vi "ReadCurrAD.vi"(6 "time out":u32, 10 "类型":u32(ring)=4 items=["PCI5121"=1, "PCI9810"=2, "USBCAN1"=3, "USBCAN2"=4, "PCI9820"=5, "CAN232"=6, "PCI5110"=7, "CANLite(mini)"=8, "ISA9620"=9, "ISA5420"=10, "PC104CAN"=11, "CANET"=17, "DNP9810"=13, "USBCAN-E-U"=20, "USBCAN-2E-U"=21], 12 "设备索引":u32(ring) items=["0", "1", "2", "3", "4", "5", "6", "7", "8", "9", "10", "11", "12", "13", "14", "15", ""], 16 "CAN路数":u32(ring) items=["0", "1"]) -> (20 "set ok?":bool, 23 "AD":u16)   [LabVIEW 2013]
uses:
  AutoBurn/Settings/ControlCAN.dll
panel:
  out "VCI_CAN_OBJ_T":T1 {"ID" format="%x"}
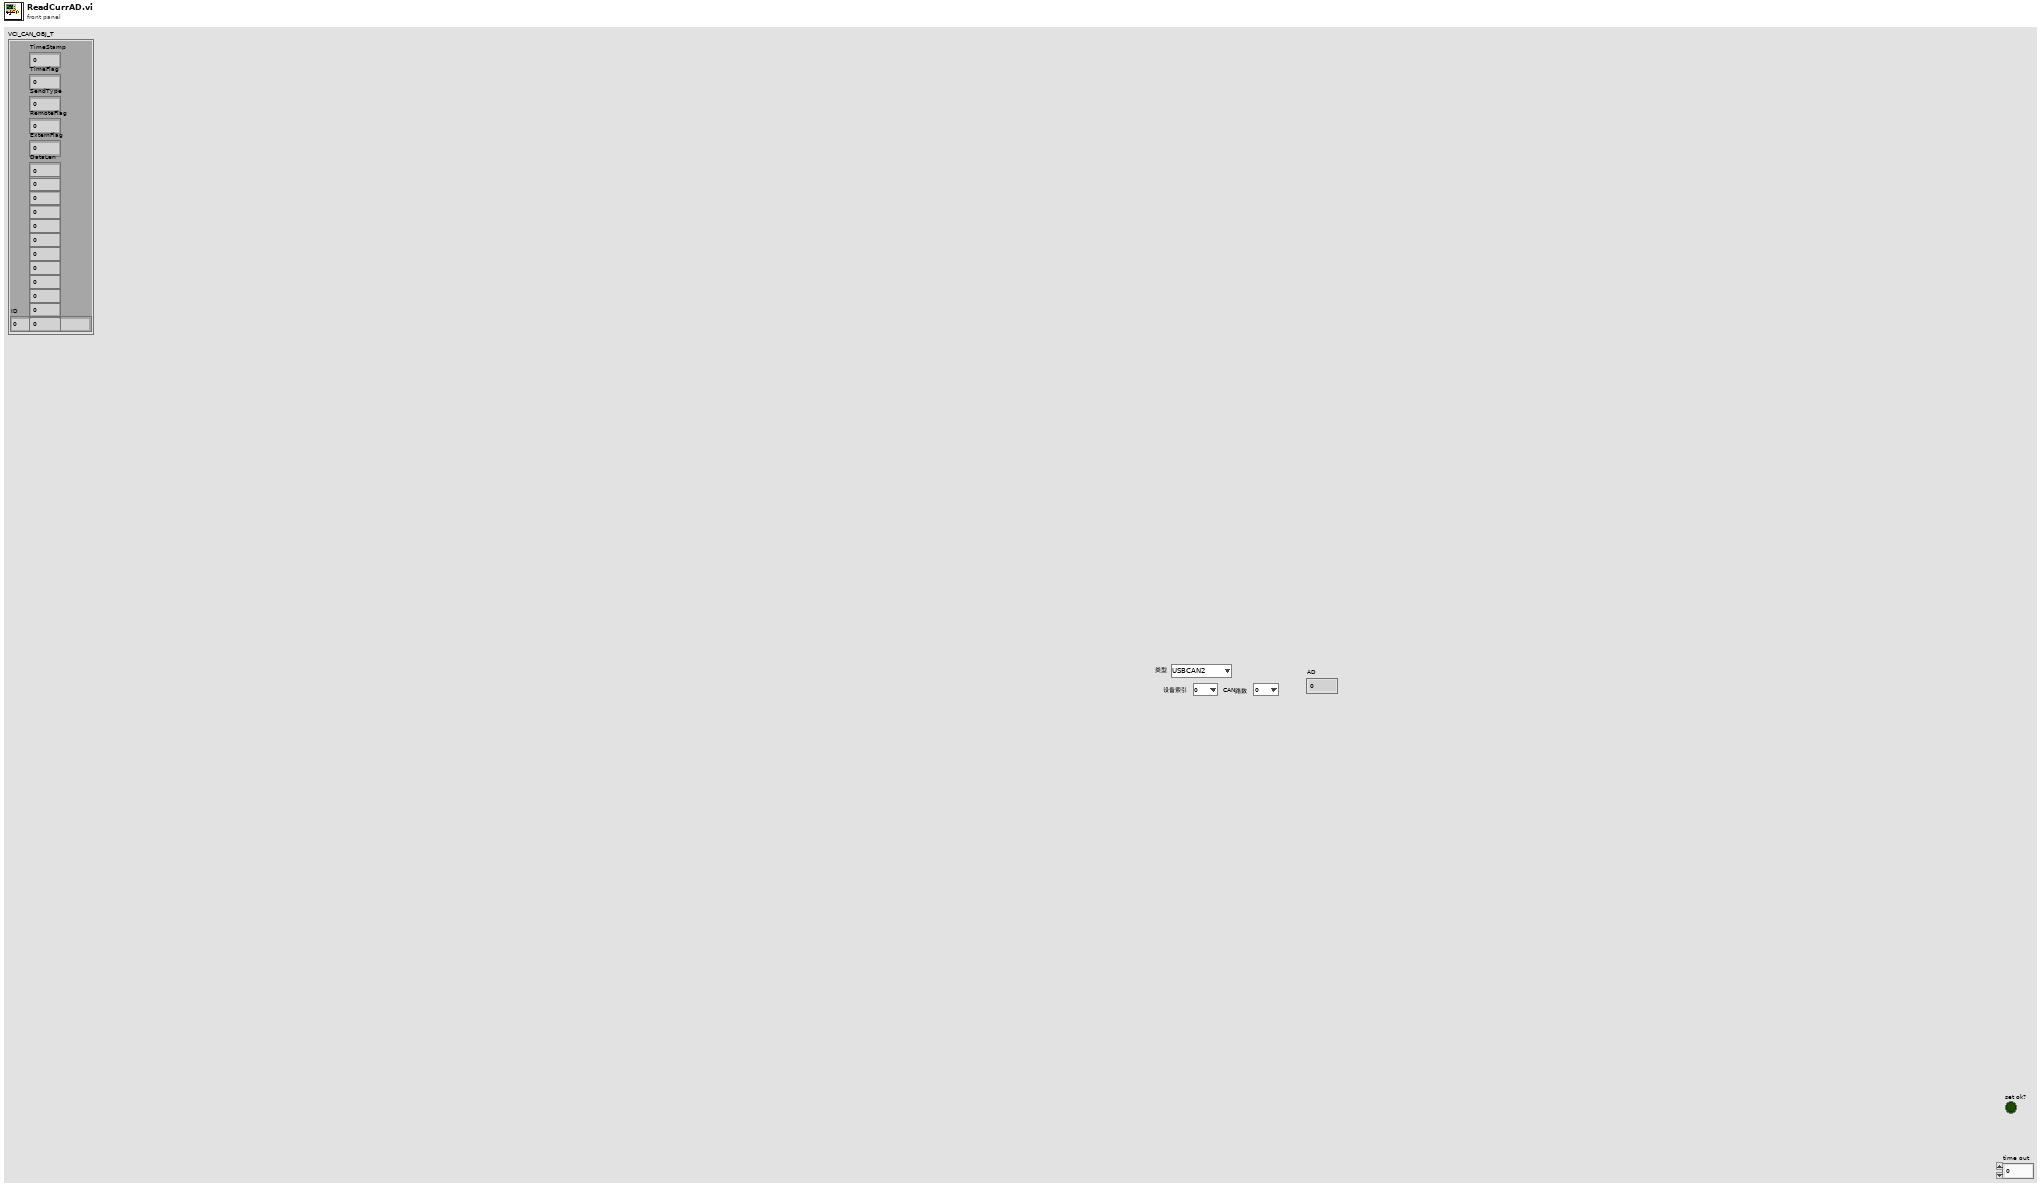
[diagram p1: front panel]
types:
  T1 = cluster{"ID":u32, "TimeStamp":u32, "TimeFlag":u8, "SendType":u8, "RemoteFlag":u8, "ExternFlag":u8, "DataLen":u8, u8, u8, u8, u8, u8, u8, u8, u8, u8, u8, u8}
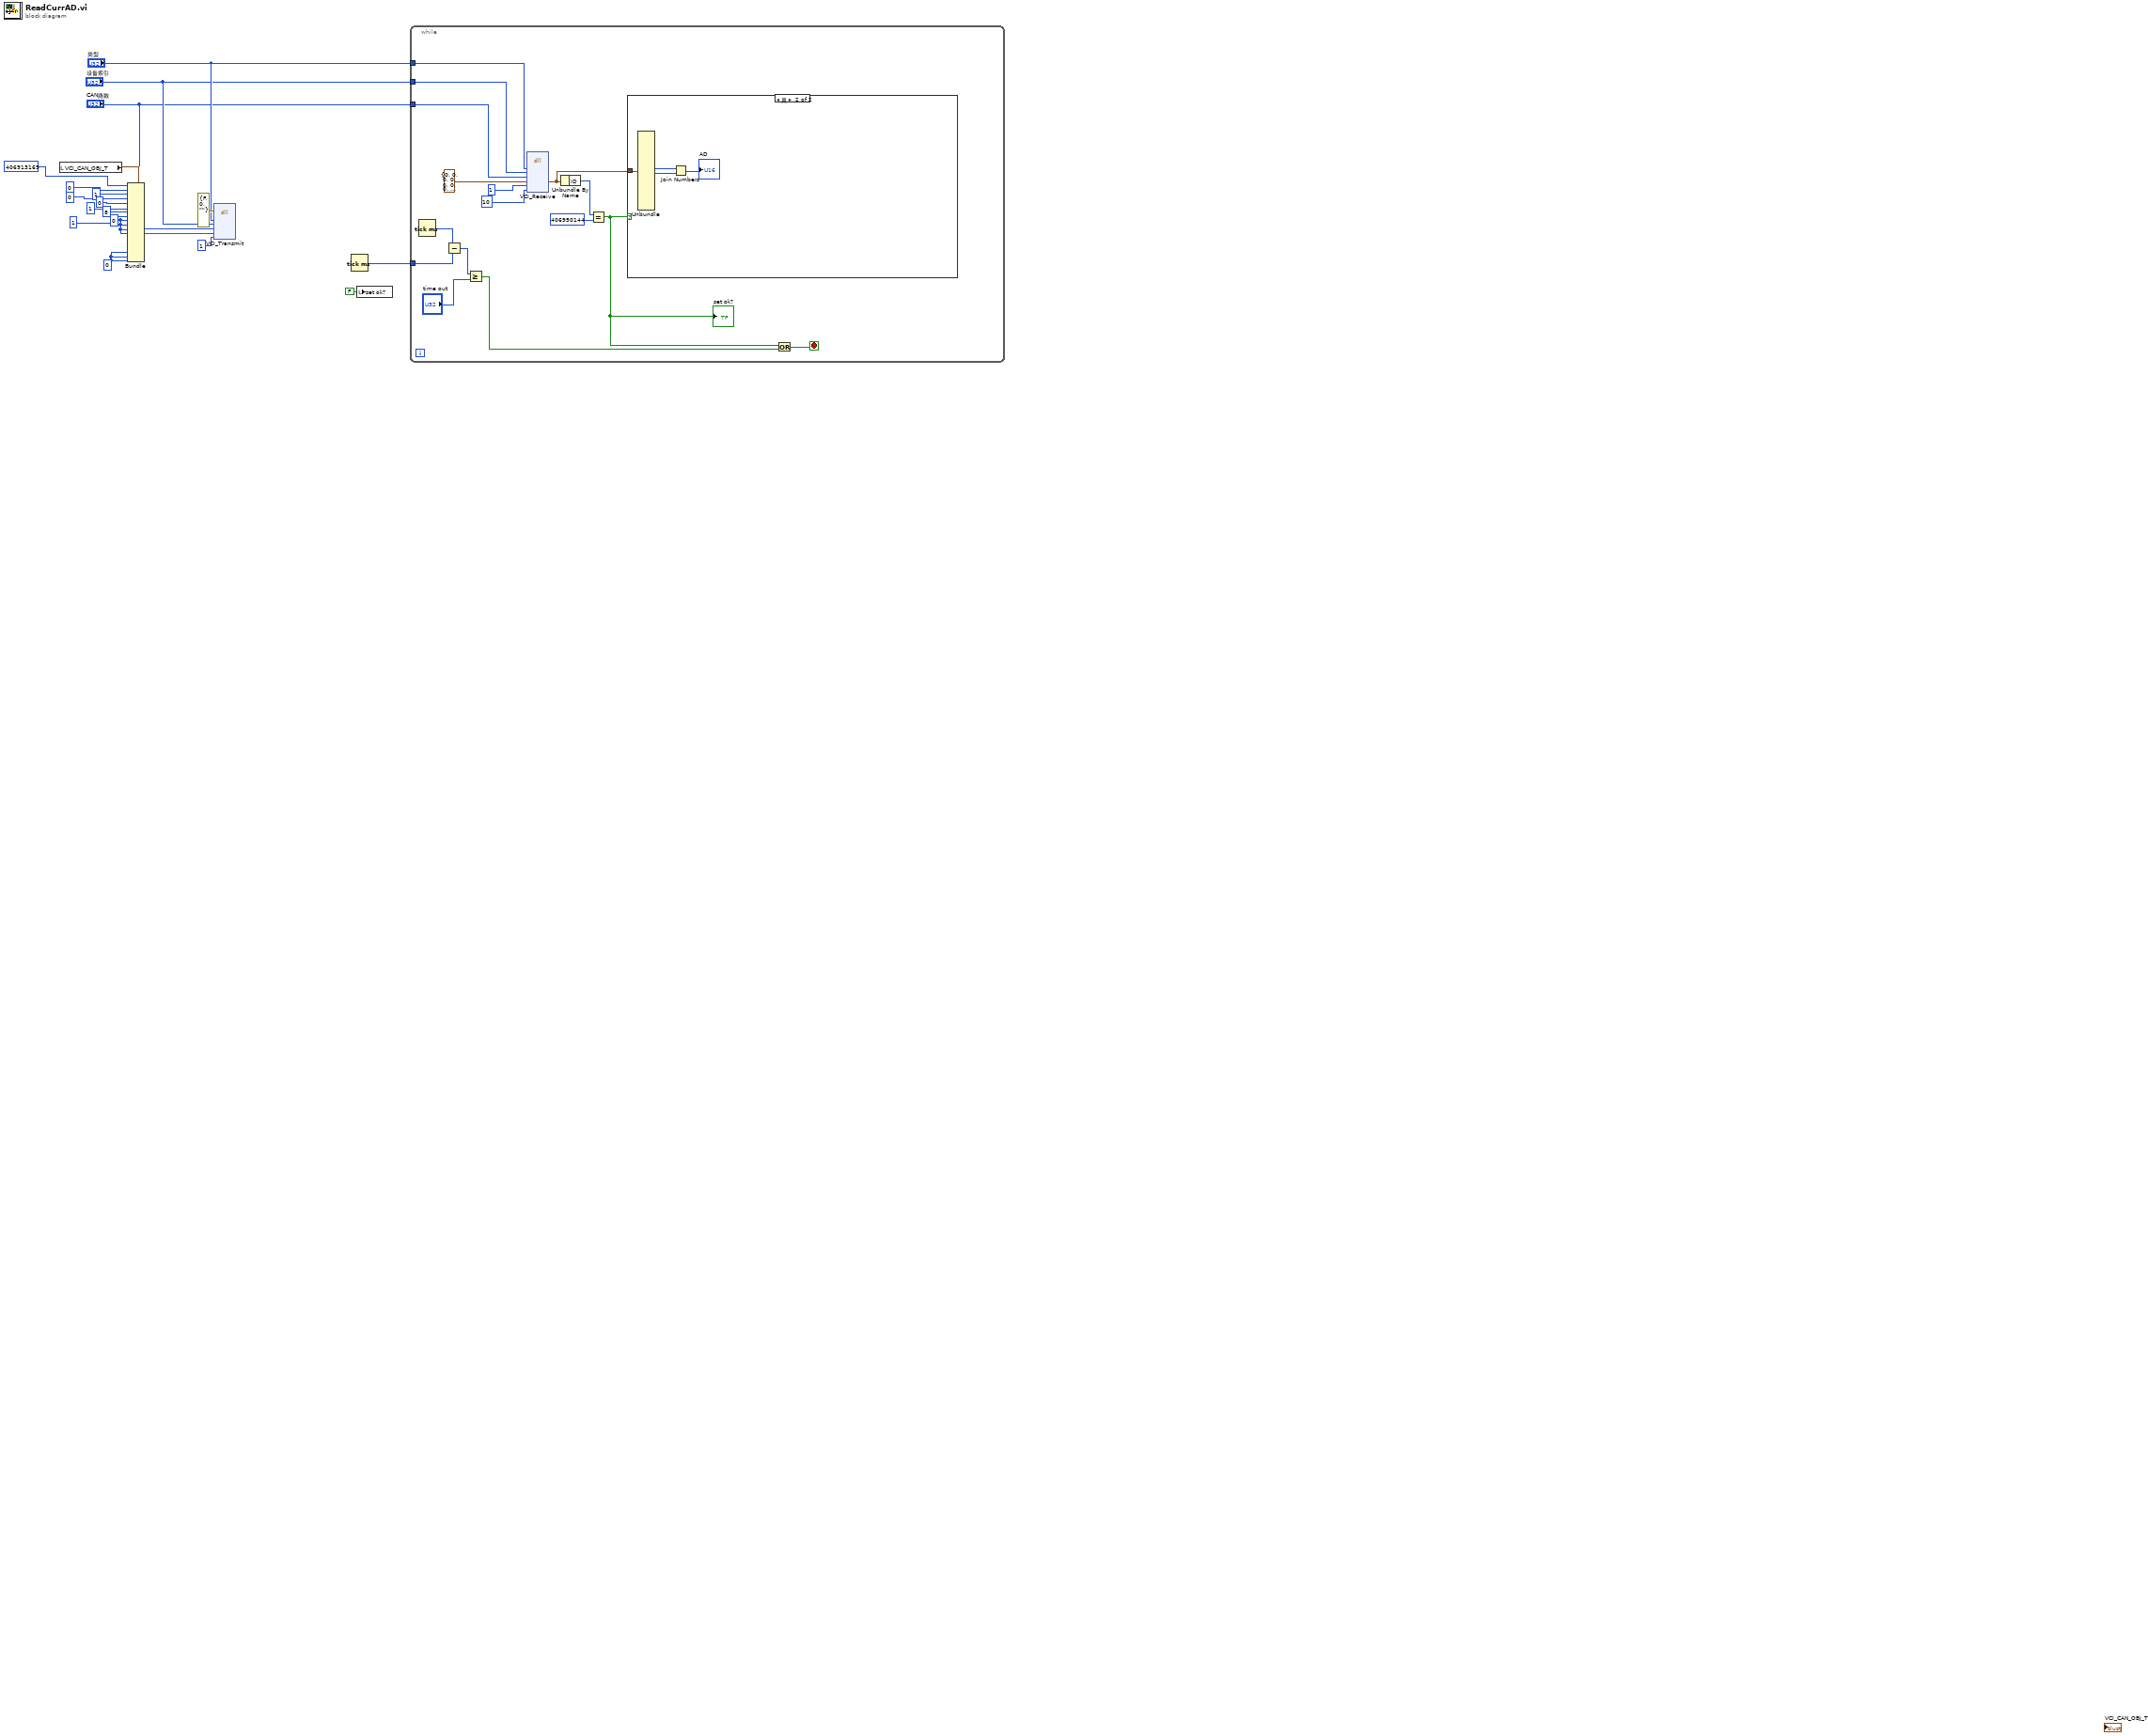
[diagram p0: block diagram]
diagram:
  w1 = u8 0
  w11 = u8 0 ("元素")
  n1 = local read "VCI_CAN_OBJ_T"() -> (w15:T1)
  n2 = Bundle(cluster=w15, "ID"=u32 406913169 ("RemoteFlag"), "TimeStamp"=u8 0 ("RemoteFlag"), "TimeFlag"=u8 1, "SendType"=u8 0 ("DataLen"), "RemoteFlag"=u8 0, "ExternFlag"=u8 1, "DataLen"=u8 8, u8 1, w1, w1, w1, w1, w11, w11, w11) -> (w16:T1)  [unwired: 3 in]
  n3 = dll-call lib="F:/Bluewave New Energy/SVN_Work/AutoTest_TestStand/trunk/AutoTest_TestStand/Driver/ZlgCan/BHN01/AutoBurn/Settings/ControlCAN.dll" fn="VCI_Transmit"(error in=errorcluster {"status"=FALSE, "code"=0, "source"=""} ("错误输入（无错误）"), "DeviceType"="类型", "DeviceInd"="设备索引", "CANInd"="CAN路数", "pSend"=w16, "Len"=u32 1) -> ()  [unwired: 4 in, 6 out]
  n4 = Tick Count (ms)() -> (millisecond timer value=w19:u32)
  n5 = local write "set ok?"(FALSE ("x = y?")) -> ()
  n6 = while {
    tunnel: w19 -> [w31]
    tunnel: "类型" -> [w23]
    tunnel: "设备索引" -> [w22]
    tunnel: "CAN路数" -> [w21]
    stop <- w26 stop-if-true
    n7 = Tick Count (ms)() -> (millisecond timer value=w32:u32)
    n8 = Subtract(x=w32, y=w31) -> (x-y=w30:u32)
    n9 = Greater Or Equal?(x=w30, y="time out") -> (x >= y?=w27:bool)
    n10 = dll-call lib="F:/Bluewave New Energy/SVN_Work/AutoTest_TestStand/trunk/AutoTest_TestStand/Driver/ZlgCan/BHN01/AutoBurn/Settings/ControlCAN.dll" fn="VCI_Receive"("DeviceType"=w23, "DeviceInd"=w22, "CANInd"=w21, "pReceive"=T1 {"ID"=0, "TimeStamp"=0, "TimeFlag"=0, "SendType"=0, "RemoteFlag"=0, "ExternFlag"=0, "DataLen"=0, 0, 0, 0, 0, 0, 0, 0, 0, 0, 0, 0}, "Len"=u32 1, "WaitTime"=10) -> ("pReceive"=w25:T1)  [unwired: 8 in, 3 out]
    n11 = Unbundle By Name(w25) -> ("ID"=w28:u32)
    n12 = Equal?(x=w28, y=u32 406950144) -> (x = y?=w20:bool)
    "set ok?" <- w20
    n13 = case shown="真" w20 {
      tunnel: w25 -> [_ w39]
      frame False {
      }
      frame True {
        n14 = Unbundle(w39) -> (w38:u8, w37:u8)  [unwired: 16 out]
        n15 = Join Numbers(hi=w38, lo=w37) -> ((hi.lo)=→"AD":u16)
      }
    }
    n16 = Or(x=w20, y=w27) -> (x .or. y?=w26:bool)
  }
